vi "prototype2.21_FM_Acute.vi"() -> ()   [LabVIEW 2011]
uses:
  <vilib>/Utility/file.llb/Write To Spreadsheet File (DBL).vi
panel:
  out "Numeric 24":dbl
  in  "Path 24":path=path "C:/Users/Nieh Lab/Documents/text.xls"
  out "Mill 24":bool
  out "Numeric 23":dbl
  in  "Path 23":path=path "C:/Users/Nieh Lab/Documents/text.xls"
  out "Mill 23":bool
  out "Numeric 22":dbl
  in  "Path 22":path=path "C:/Users/Nieh Lab/Documents/text.xls"
  out "Mill 22":bool
  out "Numeric 21":dbl
  in  "Path 21":path=path "C:/Users/Nieh Lab/Documents/text.xls"
  out "Mill 21":bool
  out "Mill 11":dbl
  in  "Path 11":path=path "C:/Users/Nieh Lab/Documents/text.xls"
  out "Mill 11":bool
  out "Mill 20":dbl
  in  "Path 20":path=path "C:/Users/Nieh Lab/Documents/text.xls"
  out "Mill 20":bool
  out "Numeric 19":dbl
  in  "Path 19":path=path "C:/Users/Nieh Lab/Documents/text.xls"
  out "Mill 19":bool
  out "Mill 18":dbl
  in  "Path 18":path=path "C:/Users/Nieh Lab/Documents/text.xls"
  out "Mill 18":bool
  out "Mill 17":dbl
  in  "Path 17":path=path "C:/Users/Nieh Lab/Documents/text.xls"
  out "Mill 17":bool
  out "Mill 16":dbl
  in  "Path 16":path=path "C:/Users/Nieh Lab/Documents/text.xls"
  out "Mill 16":bool
  out "Mill 15":dbl
  in  "Path 15":path=path "C:/Users/Nieh Lab/Documents/text.xls"
  out "Mill 15":bool
  out "Mill 14":dbl
  in  "Path 14":path=path "C:/Users/Nieh Lab/Documents/text.xls"
  out "Mill 14":bool
  out "Mill 13":dbl
  in  "Path 13":path=path "C:/Users/Nieh Lab/Documents/text.xls"
  out "Mill 13":bool
  out "Mill 12":dbl
  in  "Path 12":path=path "C:/Users/Nieh Lab/Documents/text.xls"
  out "Mill 12":bool
  out "Mill 10":dbl
  in  "Path 10":path=path "C:/Users/Nieh Lab/Documents/text.xls"
  out "Mill 10":bool
  out "Mill 9":dbl
  in  "Path 9":path=path "C:/Users/Nieh Lab/Documents/text.xls"
  out "Mill 9":bool
  out "Mill 8":dbl
  in  "Path 8":path=path "C:/Users/Nieh Lab/Documents/text.xls"
  out "Mill 8":bool
  out "Mill 7":dbl
  in  "Path 7":path=path "C:/Users/Nieh Lab/Documents/text.xls"
  out "Mill 7":bool
  out "Mill 6":dbl
  in  "Path 6":path=path "C:/Users/Nieh Lab/Documents/text.xls"
  out "Mill 6":bool
  out "Mill 5":dbl
  in  "Path 5":path=path "C:/Users/Nieh Lab/Documents/text.xls"
  out "Mill 5":bool
  out "Mill 4":dbl
  in  "Path 4":path=path "C:/Users/Nieh Lab/Documents/text.xls"
  out "Mill 4":bool
  out "Mill 3":dbl
  in  "Path 3":path=path "C:/Users/Nieh Lab/Documents/text.xls"
  out "Mill 3":bool
  out "Mill 2":dbl
  in  "Path 2":path=path "C:/Users/Nieh Lab/Documents/text.xls"
  out "Mill 2":bool
  in  "Path":path=path "C:/Users/Nieh Lab/Documents/text.xls"
  in  "wait (ms)":dbl=1.0
  out "Mill  1":dbl
  in  "stop":bool
  out "Mill 1":bool
  # "channel 1 corresponds to connection 1 (grounded on 2)\nsubsequent channels correspond to odd numbers\nso channel 2 corresponds to connection 3 (grounded on 4)"
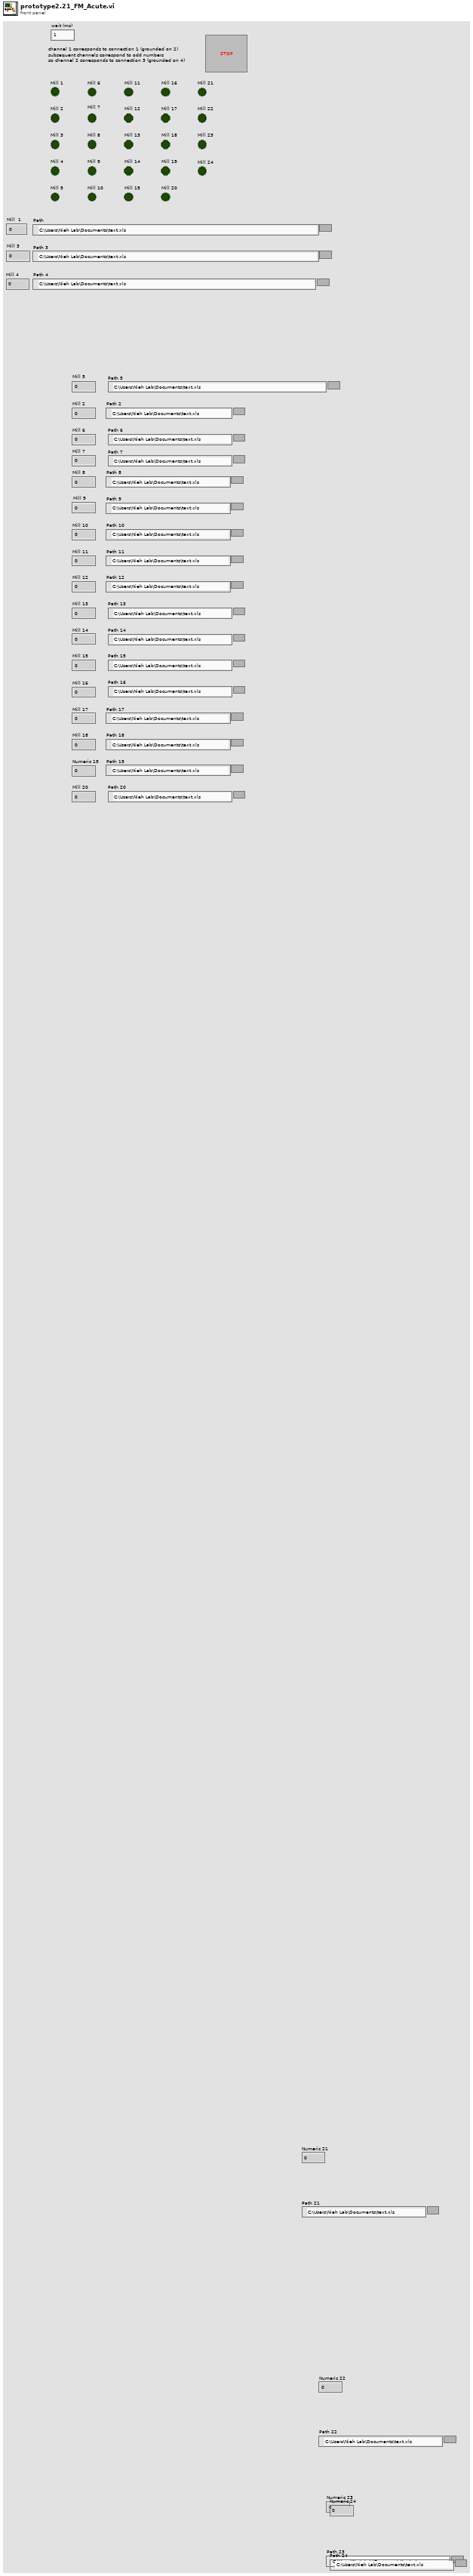
[diagram p1: front panel]
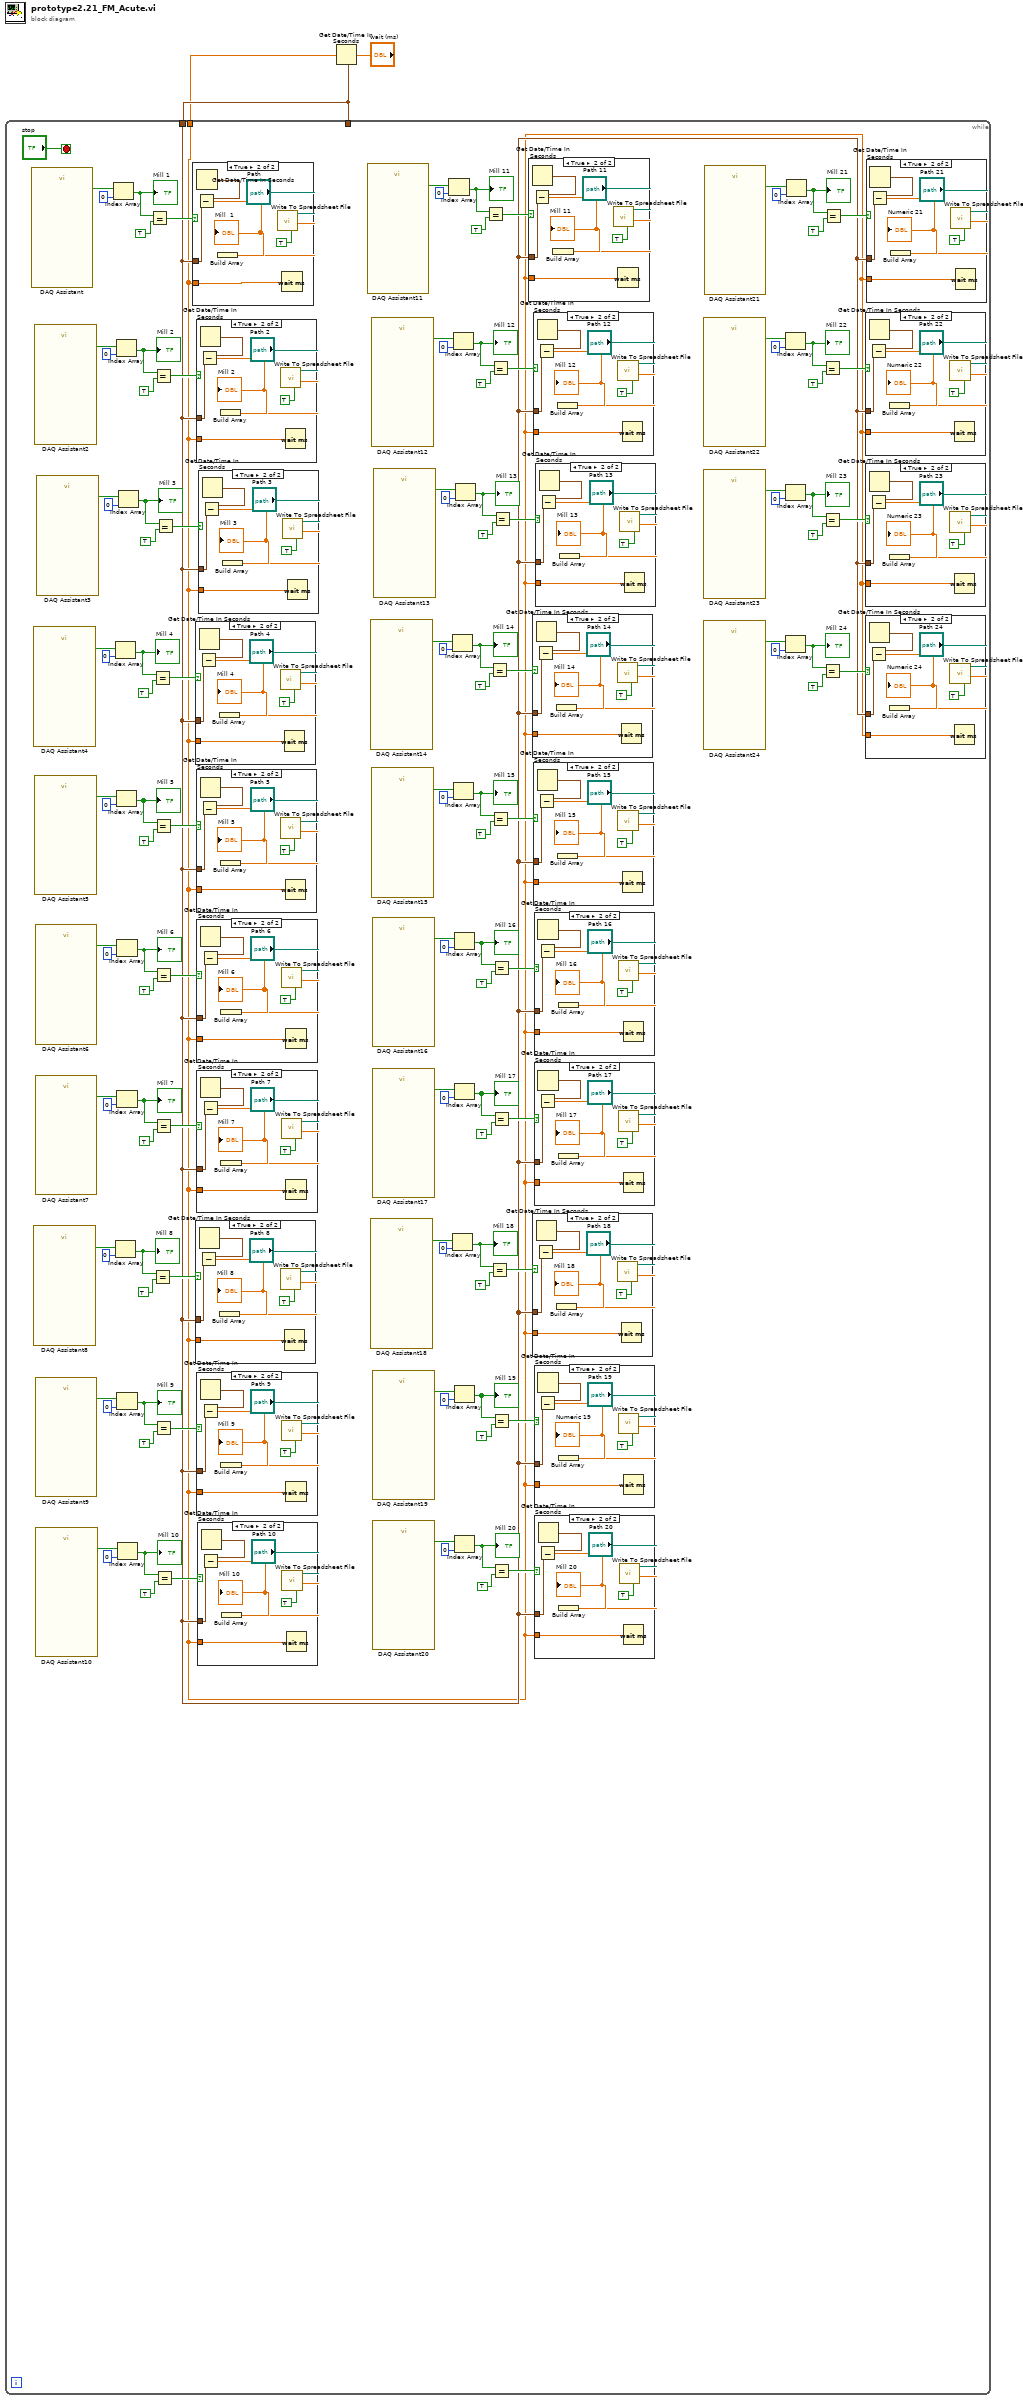
[diagram p0: block diagram]
diagram:
  n1 = Get Date/Time In Seconds() -> (seconds since 1Jan1904=w2:timestamp)
  n2 = while {
    tunnel: w2 -> [_]
    tunnel: w2 -> [w4]
    tunnel: "wait (ms)" -> [w3]
    stop <- "stop" stop-if-true
    n3 = call "DAQ Assistant"() -> ("data"=w125:bool[])  [unwired: 17 in, 2 out]
    n4 = call "DAQ Assistant4"() -> ("data"=w109:bool[])  [unwired: 17 in, 2 out]
    n5 = call "DAQ Assistant8"() -> ("data"=w89:bool[])  [unwired: 17 in, 2 out]
    n6 = call "DAQ Assistant2"() -> ("data"=w119:bool[])  [unwired: 17 in, 2 out]
    n7 = call "DAQ Assistant5"() -> ("data"=w104:bool[])  [unwired: 17 in, 2 out]
    n8 = call "DAQ Assistant6"() -> ("data"=w99:bool[])  [unwired: 17 in, 2 out]
    n9 = call "DAQ Assistant7"() -> ("data"=w94:bool[])  [unwired: 17 in, 2 out]
    n10 = call "DAQ Assistant9"() -> ("data"=w84:bool[])  [unwired: 17 in, 2 out]
    n11 = call "DAQ Assistant10"() -> ("data"=w79:bool[])  [unwired: 17 in, 2 out]
    n12 = call "DAQ Assistant3"() -> ("data"=w114:bool[])  [unwired: 17 in, 2 out]
    n13 = Index Array(array=w125, index=0) -> (element=w122:bool)
    "Mill 1" <- w122
    n14 = Index Array(array=w109, index=0) -> (element=w107:bool)
    "Mill 4" <- w107
    n15 = Index Array(array=w89, index=0) -> (element=w87:bool)
    "Mill 8" <- w87
    n16 = Index Array(array=w119, index=0) -> (element=w117:bool)
    "Mill 2" <- w117
    n17 = Index Array(array=w104, index=0) -> (element=w102:bool)
    "Mill 5" <- w102
    n18 = Index Array(array=w99, index=0) -> (element=w97:bool)
    "Mill 6" <- w97
    n19 = Index Array(array=w94, index=0) -> (element=w92:bool)
    "Mill 7" <- w92
    n20 = Index Array(array=w84, index=0) -> (element=w82:bool)
    "Mill 9" <- w82
    n21 = Index Array(array=w79, index=0) -> (element=w77:bool)
    "Mill 10" <- w77
    n22 = Index Array(array=w114, index=0) -> (element=w112:bool)
    "Mill 3" <- w112
    n23 = Equal?(x=w122, y=TRUE) -> (x = y?=w120:bool)
    n24 = Equal?(x=w107, y=TRUE) -> (x = y?=w105:bool)
    n25 = Equal?(x=w87, y=TRUE) -> (x = y?=w85:bool)
    n26 = Equal?(x=w117, y=TRUE) -> (x = y?=w115:bool)
    n27 = Equal?(x=w102, y=TRUE) -> (x = y?=w100:bool)
    n28 = Equal?(x=w97, y=TRUE) -> (x = y?=w95:bool)
    n29 = Equal?(x=w92, y=TRUE) -> (x = y?=w90:bool)
    n30 = Equal?(x=w82, y=TRUE) -> (x = y?=w80:bool)
    n31 = Equal?(x=w77, y=TRUE) -> (x = y?=w75:bool)
    n32 = Equal?(x=w112, y=TRUE) -> (x = y?=w110:bool)
    n33 = case shown="True" w120 {
      tunnel: w4 -> [_ w293]
      tunnel: w3 -> [_ w287]
      frame False {
      }
      frame True {
        n34 = Get Date/Time In Seconds() -> (seconds since 1Jan1904=w292:timestamp)
        n35 = Subtract(x=w292, y=w293) -> (x-y=w291:dbl)
        "Mill  1" <- w291
        n36 = Build Array(w291) -> (w290:dbl[])
        n37 = call-poly <vilib>:"Write To Spreadsheet File.vi"("append to file? (new file:F)"=TRUE, "1D data"=w290, "file path (dialog if empty)"="Path") -> ()  [unwired: 5 in, 1 out]
        n38 = Wait (ms)(milliseconds to wait=w287) -> ()  [unwired: 1 out]
      }
    }
    n39 = case shown="True" w105 {
      tunnel: w4 -> [_ w272]
      tunnel: w3 -> [_ w266]
      frame False {
      }
      frame True {
        n40 = Get Date/Time In Seconds() -> (seconds since 1Jan1904=w271:timestamp)
        n41 = Subtract(x=w271, y=w272) -> (x-y=w270:dbl)
        "Mill 4" <- w270
        n42 = Build Array(w270) -> (w269:dbl[])
        n43 = call-poly <vilib>:"Write To Spreadsheet File.vi"("append to file? (new file:F)"=TRUE, "1D data"=w269, "file path (dialog if empty)"="Path 4") -> ()  [unwired: 5 in, 1 out]
        n44 = Wait (ms)(milliseconds to wait=w266) -> ()  [unwired: 1 out]
      }
    }
    n45 = case shown="True" w85 {
      tunnel: w4 -> [_ w244]
      tunnel: w3 -> [_ w238]
      frame False {
      }
      frame True {
        n46 = Get Date/Time In Seconds() -> (seconds since 1Jan1904=w243:timestamp)
        n47 = Subtract(x=w243, y=w244) -> (x-y=w242:dbl)
        "Mill 8" <- w242
        n48 = Build Array(w242) -> (w241:dbl[])
        n49 = call-poly <vilib>:"Write To Spreadsheet File.vi"("append to file? (new file:F)"=TRUE, "1D data"=w241, "file path (dialog if empty)"="Path 8") -> ()  [unwired: 5 in, 1 out]
        n50 = Wait (ms)(milliseconds to wait=w238) -> ()  [unwired: 1 out]
      }
    }
    n51 = case shown="True" w115 {
      tunnel: w4 -> [_ w286]
      tunnel: w3 -> [_ w280]
      frame False {
      }
      frame True {
        n52 = Get Date/Time In Seconds() -> (seconds since 1Jan1904=w285:timestamp)
        n53 = Subtract(x=w285, y=w286) -> (x-y=w284:dbl)
        "Mill 2" <- w284
        n54 = Build Array(w284) -> (w283:dbl[])
        n55 = call-poly <vilib>:"Write To Spreadsheet File.vi"("append to file? (new file:F)"=TRUE, "1D data"=w283, "file path (dialog if empty)"="Path 2") -> ()  [unwired: 5 in, 1 out]
        n56 = Wait (ms)(milliseconds to wait=w280) -> ()  [unwired: 1 out]
      }
    }
    n57 = case shown="True" w100 {
      tunnel: w4 -> [_ w265]
      tunnel: w3 -> [_ w259]
      frame False {
      }
      frame True {
        n58 = Get Date/Time In Seconds() -> (seconds since 1Jan1904=w264:timestamp)
        n59 = Subtract(x=w264, y=w265) -> (x-y=w263:dbl)
        "Mill 5" <- w263
        n60 = Build Array(w263) -> (w262:dbl[])
        n61 = call-poly <vilib>:"Write To Spreadsheet File.vi"("append to file? (new file:F)"=TRUE, "1D data"=w262, "file path (dialog if empty)"="Path 5") -> ()  [unwired: 5 in, 1 out]
        n62 = Wait (ms)(milliseconds to wait=w259) -> ()  [unwired: 1 out]
      }
    }
    n63 = case shown="True" w95 {
      tunnel: w4 -> [_ w258]
      tunnel: w3 -> [_ w252]
      frame False {
      }
      frame True {
        n64 = Get Date/Time In Seconds() -> (seconds since 1Jan1904=w257:timestamp)
        n65 = Subtract(x=w257, y=w258) -> (x-y=w256:dbl)
        "Mill 6" <- w256
        n66 = Build Array(w256) -> (w255:dbl[])
        n67 = call-poly <vilib>:"Write To Spreadsheet File.vi"("append to file? (new file:F)"=TRUE, "1D data"=w255, "file path (dialog if empty)"="Path 6") -> ()  [unwired: 5 in, 1 out]
        n68 = Wait (ms)(milliseconds to wait=w252) -> ()  [unwired: 1 out]
      }
    }
    n69 = case shown="True" w90 {
      tunnel: w4 -> [_ w251]
      tunnel: w3 -> [_ w245]
      frame False {
      }
      frame True {
        n70 = Get Date/Time In Seconds() -> (seconds since 1Jan1904=w250:timestamp)
        n71 = Subtract(x=w250, y=w251) -> (x-y=w249:dbl)
        "Mill 7" <- w249
        n72 = Build Array(w249) -> (w248:dbl[])
        n73 = call-poly <vilib>:"Write To Spreadsheet File.vi"("append to file? (new file:F)"=TRUE, "1D data"=w248, "file path (dialog if empty)"="Path 7") -> ()  [unwired: 5 in, 1 out]
        n74 = Wait (ms)(milliseconds to wait=w245) -> ()  [unwired: 1 out]
      }
    }
    n75 = case shown="True" w80 {
      tunnel: w4 -> [_ w237]
      tunnel: w3 -> [_ w231]
      frame False {
      }
      frame True {
        n76 = Get Date/Time In Seconds() -> (seconds since 1Jan1904=w236:timestamp)
        n77 = Subtract(x=w236, y=w237) -> (x-y=w235:dbl)
        "Mill 9" <- w235
        n78 = Build Array(w235) -> (w234:dbl[])
        n79 = call-poly <vilib>:"Write To Spreadsheet File.vi"("append to file? (new file:F)"=TRUE, "1D data"=w234, "file path (dialog if empty)"="Path 9") -> ()  [unwired: 5 in, 1 out]
        n80 = Wait (ms)(milliseconds to wait=w231) -> ()  [unwired: 1 out]
      }
    }
    n81 = case shown="True" w75 {
      tunnel: w4 -> [_ w230]
      tunnel: w3 -> [_ w224]
      frame False {
      }
      frame True {
        n82 = Get Date/Time In Seconds() -> (seconds since 1Jan1904=w229:timestamp)
        n83 = Subtract(x=w229, y=w230) -> (x-y=w228:dbl)
        "Mill 10" <- w228
        n84 = Build Array(w228) -> (w227:dbl[])
        n85 = call-poly <vilib>:"Write To Spreadsheet File.vi"("append to file? (new file:F)"=TRUE, "1D data"=w227, "file path (dialog if empty)"="Path 10") -> ()  [unwired: 5 in, 1 out]
        n86 = Wait (ms)(milliseconds to wait=w224) -> ()  [unwired: 1 out]
      }
    }
    n87 = case shown="True" w110 {
      tunnel: w4 -> [_ w279]
      tunnel: w3 -> [_ w273]
      frame False {
      }
      frame True {
        n88 = Get Date/Time In Seconds() -> (seconds since 1Jan1904=w278:timestamp)
        n89 = Subtract(x=w278, y=w279) -> (x-y=w277:dbl)
        "Mill 3" <- w277
        n90 = Build Array(w277) -> (w276:dbl[])
        n91 = call-poly <vilib>:"Write To Spreadsheet File.vi"("append to file? (new file:F)"=TRUE, "1D data"=w276, "file path (dialog if empty)"="Path 3") -> ()  [unwired: 5 in, 1 out]
        n92 = Wait (ms)(milliseconds to wait=w273) -> ()  [unwired: 1 out]
      }
    }
    n93 = call "DAQ Assistant11"() -> ("data"=w29:bool[])  [unwired: 17 in, 2 out]
    n94 = call "DAQ Assistant14"() -> ("data"=w64:bool[])  [unwired: 17 in, 2 out]
    n95 = call "DAQ Assistant18"() -> ("data"=w44:bool[])  [unwired: 17 in, 2 out]
    n96 = call "DAQ Assistant12"() -> ("data"=w74:bool[])  [unwired: 17 in, 2 out]
    n97 = call "DAQ Assistant15"() -> ("data"=w59:bool[])  [unwired: 17 in, 2 out]
    n98 = call "DAQ Assistant16"() -> ("data"=w54:bool[])  [unwired: 17 in, 2 out]
    n99 = call "DAQ Assistant17"() -> ("data"=w49:bool[])  [unwired: 17 in, 2 out]
    n100 = call "DAQ Assistant19"() -> ("data"=w39:bool[])  [unwired: 17 in, 2 out]
    n101 = call "DAQ Assistant20"() -> ("data"=w34:bool[])  [unwired: 17 in, 2 out]
    n102 = call "DAQ Assistant13"() -> ("data"=w69:bool[])  [unwired: 17 in, 2 out]
    n103 = Index Array(array=w29, index=0) -> (element=w27:bool)
    "Mill 11" <- w27
    n104 = Index Array(array=w64, index=0) -> (element=w62:bool)
    "Mill 14" <- w62
    n105 = Index Array(array=w44, index=0) -> (element=w42:bool)
    "Mill 18" <- w42
    n106 = Index Array(array=w74, index=0) -> (element=w72:bool)
    "Mill 12" <- w72
    n107 = Index Array(array=w59, index=0) -> (element=w57:bool)
    "Mill 15" <- w57
    n108 = Index Array(array=w54, index=0) -> (element=w52:bool)
    "Mill 16" <- w52
    n109 = Index Array(array=w49, index=0) -> (element=w47:bool)
    "Mill 17" <- w47
    n110 = Index Array(array=w39, index=0) -> (element=w37:bool)
    "Mill 19" <- w37
    n111 = Index Array(array=w34, index=0) -> (element=w32:bool)
    "Mill 20" <- w32
    n112 = Index Array(array=w69, index=0) -> (element=w67:bool)
    "Mill 13" <- w67
    n113 = Equal?(x=w27, y=TRUE) -> (x = y?=w25:bool)
    n114 = Equal?(x=w62, y=TRUE) -> (x = y?=w60:bool)
    n115 = Equal?(x=w42, y=TRUE) -> (x = y?=w40:bool)
    n116 = Equal?(x=w72, y=TRUE) -> (x = y?=w70:bool)
    n117 = Equal?(x=w57, y=TRUE) -> (x = y?=w55:bool)
    n118 = Equal?(x=w52, y=TRUE) -> (x = y?=w50:bool)
    n119 = Equal?(x=w47, y=TRUE) -> (x = y?=w45:bool)
    n120 = Equal?(x=w37, y=TRUE) -> (x = y?=w35:bool)
    n121 = Equal?(x=w32, y=TRUE) -> (x = y?=w30:bool)
    n122 = Equal?(x=w67, y=TRUE) -> (x = y?=w65:bool)
    n123 = case shown="True" w25 {
      tunnel: w4 -> [_ w160]
      tunnel: w3 -> [_ w154]
      frame False {
      }
      frame True {
        n124 = Get Date/Time In Seconds() -> (seconds since 1Jan1904=w159:timestamp)
        n125 = Subtract(x=w159, y=w160) -> (x-y=w158:dbl)
        "Mill 11" <- w158
        n126 = Build Array(w158) -> (w157:dbl[])
        n127 = call-poly <vilib>:"Write To Spreadsheet File.vi"("append to file? (new file:F)"=TRUE, "1D data"=w157, "file path (dialog if empty)"="Path 11") -> ()  [unwired: 5 in, 1 out]
        n128 = Wait (ms)(milliseconds to wait=w154) -> ()  [unwired: 1 out]
      }
    }
    n129 = case shown="True" w60 {
      tunnel: w4 -> [_ w209]
      tunnel: w3 -> [_ w203]
      frame False {
      }
      frame True {
        n130 = Get Date/Time In Seconds() -> (seconds since 1Jan1904=w208:timestamp)
        n131 = Subtract(x=w208, y=w209) -> (x-y=w207:dbl)
        "Mill 14" <- w207
        n132 = Build Array(w207) -> (w206:dbl[])
        n133 = call-poly <vilib>:"Write To Spreadsheet File.vi"("append to file? (new file:F)"=TRUE, "1D data"=w206, "file path (dialog if empty)"="Path 14") -> ()  [unwired: 5 in, 1 out]
        n134 = Wait (ms)(milliseconds to wait=w203) -> ()  [unwired: 1 out]
      }
    }
    n135 = case shown="True" w40 {
      tunnel: w4 -> [_ w181]
      tunnel: w3 -> [_ w175]
      frame False {
      }
      frame True {
        n136 = Get Date/Time In Seconds() -> (seconds since 1Jan1904=w180:timestamp)
        n137 = Subtract(x=w180, y=w181) -> (x-y=w179:dbl)
        "Mill 18" <- w179
        n138 = Build Array(w179) -> (w178:dbl[])
        n139 = call-poly <vilib>:"Write To Spreadsheet File.vi"("append to file? (new file:F)"=TRUE, "1D data"=w178, "file path (dialog if empty)"="Path 18") -> ()  [unwired: 5 in, 1 out]
        n140 = Wait (ms)(milliseconds to wait=w175) -> ()  [unwired: 1 out]
      }
    }
    n141 = case shown="True" w70 {
      tunnel: w4 -> [_ w223]
      tunnel: w3 -> [_ w217]
      frame False {
      }
      frame True {
        n142 = Get Date/Time In Seconds() -> (seconds since 1Jan1904=w222:timestamp)
        n143 = Subtract(x=w222, y=w223) -> (x-y=w221:dbl)
        "Mill 12" <- w221
        n144 = Build Array(w221) -> (w220:dbl[])
        n145 = call-poly <vilib>:"Write To Spreadsheet File.vi"("append to file? (new file:F)"=TRUE, "1D data"=w220, "file path (dialog if empty)"="Path 12") -> ()  [unwired: 5 in, 1 out]
        n146 = Wait (ms)(milliseconds to wait=w217) -> ()  [unwired: 1 out]
      }
    }
    n147 = case shown="True" w55 {
      tunnel: w4 -> [_ w202]
      tunnel: w3 -> [_ w196]
      frame False {
      }
      frame True {
        n148 = Get Date/Time In Seconds() -> (seconds since 1Jan1904=w201:timestamp)
        n149 = Subtract(x=w201, y=w202) -> (x-y=w200:dbl)
        "Mill 15" <- w200
        n150 = Build Array(w200) -> (w199:dbl[])
        n151 = call-poly <vilib>:"Write To Spreadsheet File.vi"("append to file? (new file:F)"=TRUE, "1D data"=w199, "file path (dialog if empty)"="Path 15") -> ()  [unwired: 5 in, 1 out]
        n152 = Wait (ms)(milliseconds to wait=w196) -> ()  [unwired: 1 out]
      }
    }
    n153 = case shown="True" w50 {
      tunnel: w4 -> [_ w195]
      tunnel: w3 -> [_ w189]
      frame False {
      }
      frame True {
        n154 = Get Date/Time In Seconds() -> (seconds since 1Jan1904=w194:timestamp)
        n155 = Subtract(x=w194, y=w195) -> (x-y=w193:dbl)
        "Mill 16" <- w193
        n156 = Build Array(w193) -> (w192:dbl[])
        n157 = call-poly <vilib>:"Write To Spreadsheet File.vi"("append to file? (new file:F)"=TRUE, "1D data"=w192, "file path (dialog if empty)"="Path 16") -> ()  [unwired: 5 in, 1 out]
        n158 = Wait (ms)(milliseconds to wait=w189) -> ()  [unwired: 1 out]
      }
    }
    n159 = case shown="True" w45 {
      tunnel: w4 -> [_ w188]
      tunnel: w3 -> [_ w182]
      frame False {
      }
      frame True {
        n160 = Get Date/Time In Seconds() -> (seconds since 1Jan1904=w187:timestamp)
        n161 = Subtract(x=w187, y=w188) -> (x-y=w186:dbl)
        "Mill 17" <- w186
        n162 = Build Array(w186) -> (w185:dbl[])
        n163 = call-poly <vilib>:"Write To Spreadsheet File.vi"("append to file? (new file:F)"=TRUE, "1D data"=w185, "file path (dialog if empty)"="Path 17") -> ()  [unwired: 5 in, 1 out]
        n164 = Wait (ms)(milliseconds to wait=w182) -> ()  [unwired: 1 out]
      }
    }
    n165 = case shown="True" w35 {
      tunnel: w4 -> [_ w174]
      tunnel: w3 -> [_ w168]
      frame False {
      }
      frame True {
        n166 = Get Date/Time In Seconds() -> (seconds since 1Jan1904=w173:timestamp)
        n167 = Subtract(x=w173, y=w174) -> (x-y=w172:dbl)
        "Numeric 19" <- w172
        n168 = Build Array(w172) -> (w171:dbl[])
        n169 = call-poly <vilib>:"Write To Spreadsheet File.vi"("append to file? (new file:F)"=TRUE, "1D data"=w171, "file path (dialog if empty)"="Path 19") -> ()  [unwired: 5 in, 1 out]
        n170 = Wait (ms)(milliseconds to wait=w168) -> ()  [unwired: 1 out]
      }
    }
    n171 = case shown="True" w30 {
      tunnel: w4 -> [_ w167]
      tunnel: w3 -> [_ w161]
      frame False {
      }
      frame True {
        n172 = Get Date/Time In Seconds() -> (seconds since 1Jan1904=w166:timestamp)
        n173 = Subtract(x=w166, y=w167) -> (x-y=w165:dbl)
        "Mill 20" <- w165
        n174 = Build Array(w165) -> (w164:dbl[])
        n175 = call-poly <vilib>:"Write To Spreadsheet File.vi"("append to file? (new file:F)"=TRUE, "1D data"=w164, "file path (dialog if empty)"="Path 20") -> ()  [unwired: 5 in, 1 out]
        n176 = Wait (ms)(milliseconds to wait=w161) -> ()  [unwired: 1 out]
      }
    }
    n177 = case shown="True" w65 {
      tunnel: w4 -> [_ w216]
      tunnel: w3 -> [_ w210]
      frame False {
      }
      frame True {
        n178 = Get Date/Time In Seconds() -> (seconds since 1Jan1904=w215:timestamp)
        n179 = Subtract(x=w215, y=w216) -> (x-y=w214:dbl)
        "Mill 13" <- w214
        n180 = Build Array(w214) -> (w213:dbl[])
        n181 = call-poly <vilib>:"Write To Spreadsheet File.vi"("append to file? (new file:F)"=TRUE, "1D data"=w213, "file path (dialog if empty)"="Path 13") -> ()  [unwired: 5 in, 1 out]
        n182 = Wait (ms)(milliseconds to wait=w210) -> ()  [unwired: 1 out]
      }
    }
    n183 = call "DAQ Assistant22"() -> ("data"=w19:bool[])  [unwired: 17 in, 2 out]
    n184 = call "DAQ Assistant23"() -> ("data"=w14:bool[])  [unwired: 17 in, 2 out]
    n185 = call "DAQ Assistant24"() -> ("data"=w9:bool[])  [unwired: 17 in, 2 out]
    n186 = call "DAQ Assistant21"() -> ("data"=w24:bool[])  [unwired: 17 in, 2 out]
    n187 = Index Array(array=w19, index=0) -> (element=w17:bool)
    "Mill 22" <- w17
    n188 = Index Array(array=w14, index=0) -> (element=w12:bool)
    "Mill 23" <- w12
    n189 = Index Array(array=w9, index=0) -> (element=w7:bool)
    "Mill 24" <- w7
    n190 = Index Array(array=w24, index=0) -> (element=w22:bool)
    "Mill 21" <- w22
    n191 = Equal?(x=w17, y=TRUE) -> (x = y?=w15:bool)
    n192 = Equal?(x=w12, y=TRUE) -> (x = y?=w10:bool)
    n193 = Equal?(x=w7, y=TRUE) -> (x = y?=w5:bool)
    n194 = Equal?(x=w22, y=TRUE) -> (x = y?=w20:bool)
    n195 = case shown="True" w15 {
      tunnel: w4 -> [_ w146]
      tunnel: w3 -> [_ w140]
      frame False {
      }
      frame True {
        n196 = Get Date/Time In Seconds() -> (seconds since 1Jan1904=w145:timestamp)
        n197 = Subtract(x=w145, y=w146) -> (x-y=w144:dbl)
        "Numeric 22" <- w144
        n198 = Build Array(w144) -> (w143:dbl[])
        n199 = call-poly <vilib>:"Write To Spreadsheet File.vi"("append to file? (new file:F)"=TRUE, "1D data"=w143, "file path (dialog if empty)"="Path 22") -> ()  [unwired: 5 in, 1 out]
        n200 = Wait (ms)(milliseconds to wait=w140) -> ()  [unwired: 1 out]
      }
    }
    n201 = case shown="True" w10 {
      tunnel: w4 -> [_ w139]
      tunnel: w3 -> [_ w133]
      frame False {
      }
      frame True {
        n202 = Get Date/Time In Seconds() -> (seconds since 1Jan1904=w138:timestamp)
        n203 = Subtract(x=w138, y=w139) -> (x-y=w137:dbl)
        "Numeric 23" <- w137
        n204 = Build Array(w137) -> (w136:dbl[])
        n205 = call-poly <vilib>:"Write To Spreadsheet File.vi"("append to file? (new file:F)"=TRUE, "1D data"=w136, "file path (dialog if empty)"="Path 23") -> ()  [unwired: 5 in, 1 out]
        n206 = Wait (ms)(milliseconds to wait=w133) -> ()  [unwired: 1 out]
      }
    }
    n207 = case shown="True" w5 {
      tunnel: w4 -> [_ w132]
      tunnel: w3 -> [_ w126]
      frame False {
      }
      frame True {
        n208 = Get Date/Time In Seconds() -> (seconds since 1Jan1904=w131:timestamp)
        n209 = Subtract(x=w131, y=w132) -> (x-y=w130:dbl)
        "Numeric 24" <- w130
        n210 = Build Array(w130) -> (w129:dbl[])
        n211 = call-poly <vilib>:"Write To Spreadsheet File.vi"("append to file? (new file:F)"=TRUE, "1D data"=w129, "file path (dialog if empty)"="Path 24") -> ()  [unwired: 5 in, 1 out]
        n212 = Wait (ms)(milliseconds to wait=w126) -> ()  [unwired: 1 out]
      }
    }
    n213 = case shown="True" w20 {
      tunnel: w4 -> [_ w153]
      tunnel: w3 -> [_ w147]
      frame False {
      }
      frame True {
        n214 = Get Date/Time In Seconds() -> (seconds since 1Jan1904=w152:timestamp)
        n215 = Subtract(x=w152, y=w153) -> (x-y=w151:dbl)
        "Numeric 21" <- w151
        n216 = Build Array(w151) -> (w150:dbl[])
        n217 = call-poly <vilib>:"Write To Spreadsheet File.vi"("append to file? (new file:F)"=TRUE, "1D data"=w150, "file path (dialog if empty)"="Path 21") -> ()  [unwired: 5 in, 1 out]
        n218 = Wait (ms)(milliseconds to wait=w147) -> ()  [unwired: 1 out]
      }
    }
  }
